vi "Test - Waveform Subtype Enum.vi"() -> ()   [LabVIEW 2013]
uses:
  source/library/Waveform Subtype Enum.ctl
panel:
  out "Null":T1 format="%.0x"
  out "Complex Single":T1 format="%.0x"
  out "Complex Double":T1 format="%.0x"
  out "Complex Extended":T1 format="%.0x"
  out "Analog U8":T1 format="%.0x"
  out "Analog U16":T1 format="%.0x"
  out "Analog U32":T1 format="%.0x"
  out "Analog U64":T1 format="%.0x"
  out "Analog I64":T1 format="%.0x"
  out "Analog I8":T1 format="%.0x"
  out "Analog I16":T1 format="%.0x"
  out "Analog I32":T1 format="%.0x"
  out "Digital Data":T1 format="%.0x"
  out "Digital Waveform":T1 format="%.0x"
  out "Dynamic Data":T1 format="%.0x"
  out "Analog Extended":T1 format="%.0x"
  out "Analog Double":T1 format="%.0x"
  out "Analog Single":T1 format="%.0x"
  out "Timestamp":T1 format="%.0x"
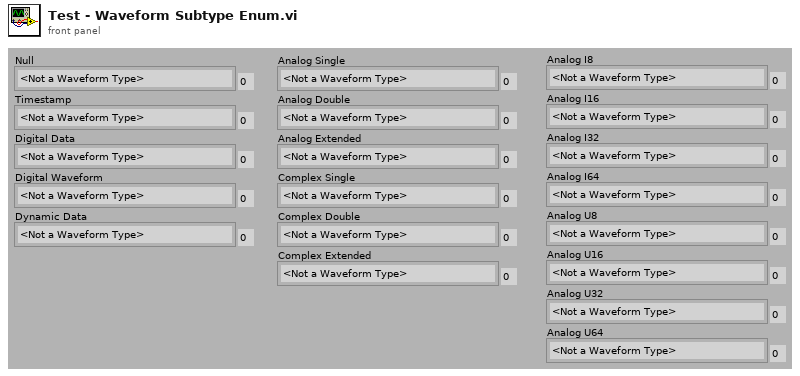
[diagram p1: front panel]
types:
  T1 = typedef "Waveform Subtype Enum.ctl" = enum8{"<Not a Waveform Type>", "0x01", "Analog 16-bit signed", "Analog Double-Precision", "0x04", "Analog Single Precision", "Timestamp", "Digital Data", "Digital Waveform", "Dynamic Data", "Analog Extended-Precision", "Analog 8-bit unsigned", "Analog 16-bit unsigned", "Analog 32-bit unsigned", "Analog 8-bit signed", "Analog 32-bit signed", "Analog Complex Single-Precision", "Analog Complex Double-Precision", "Analog Complex Extended Precision", "Analog 64-bit signed", "Analog 64-bit unsigned"}
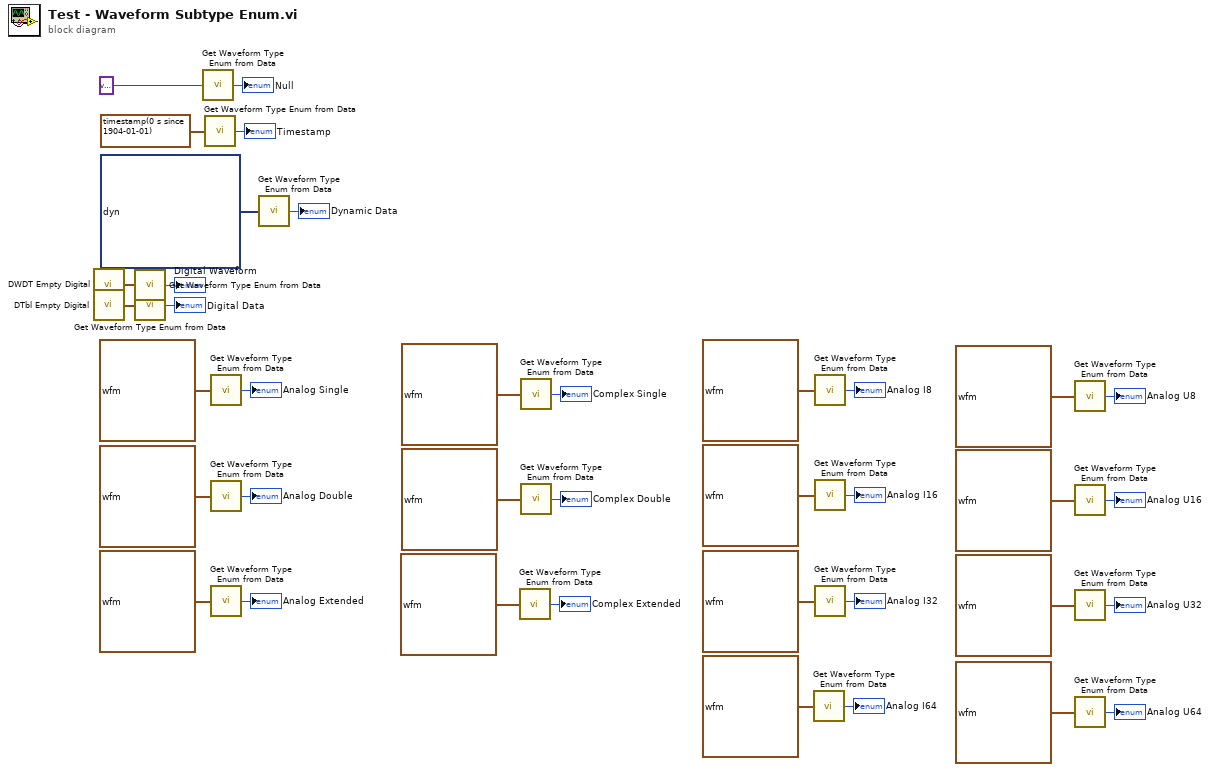
[diagram p0: block diagram]
diagram:
  n1 = call <vilib>:"DWDT Empty Digital.vi"() -> ("digital waveform out"=w27:digitalwaveform)  [unwired: 5 in]
  n2 = call <vilib>:"DTbl Empty Digital.vi"() -> ("digital data"=w25:digitaldata)  [unwired: 5 in]
  n3 = call "Get Waveform Type Enum from Data.vi"("Data"=w27) -> ("Waveform Subtype Enum"=→"Digital Waveform":T1)  [unwired: 4 in]
  n4 = call "Get Waveform Type Enum from Data.vi"("Data"=w25) -> ("Waveform Subtype Enum"=→"Digital Data":T1)  [unwired: 4 in]
  n5 = call "Get Waveform Type Enum from Data.vi"("Data"=variant ("variant")) -> ("Waveform Subtype Enum"=→"Null":T1)  [unwired: 4 in]
  n6 = call "Get Waveform Type Enum from Data.vi"("Data"=timestamp(0 s since 1904-01-01) ("Time Stamp")) -> ("Waveform Subtype Enum"=→"Timestamp":T1)  [unwired: 4 in]
  n7 = call "Get Waveform Type Enum from Data.vi"("Data"=waveform(sgl) {"t0"=timestamp(0 s since 1904-01-01), "dt"=1.0, "Y"=[]} ("waveform")) -> ("Waveform Subtype Enum"=→"Analog Single":T1)  [unwired: 4 in]
  n8 = call "Get Waveform Type Enum from Data.vi"("Data"=waveform(dbl) {"t0"=timestamp(0 s since 1904-01-01), "dt"=1.0, "Y"=[]} ("waveform")) -> ("Waveform Subtype Enum"=→"Analog Double":T1)  [unwired: 4 in]
  n9 = call "Get Waveform Type Enum from Data.vi"("Data"=waveform(ext) {"t0"=timestamp(0 s since 1904-01-01), "dt"=1.0, "Y"=[]} ("waveform")) -> ("Waveform Subtype Enum"=→"Analog Extended":T1)  [unwired: 4 in]
  n10 = call "Get Waveform Type Enum from Data.vi"("Data"=dynamicdata [] ("Waveform Graph")) -> ("Waveform Subtype Enum"=→"Dynamic Data":T1)  [unwired: 4 in]
  n11 = call "Get Waveform Type Enum from Data.vi"("Data"=waveform(cxt) {"t0"=timestamp(0 s since 1904-01-01), "dt"=1.0, "Y"=[]} ("waveform")) -> ("Waveform Subtype Enum"=→"Complex Extended":T1)  [unwired: 4 in]
  n12 = call "Get Waveform Type Enum from Data.vi"("Data"=waveform(csg) {"t0"=timestamp(0 s since 1904-01-01), "dt"=1.0, "Y"=[]} ("waveform")) -> ("Waveform Subtype Enum"=→"Complex Single":T1)  [unwired: 4 in]
  n13 = call "Get Waveform Type Enum from Data.vi"("Data"=waveform(cdb) {"t0"=timestamp(0 s since 1904-01-01), "dt"=1.0, "Y"=[]} ("waveform")) -> ("Waveform Subtype Enum"=→"Complex Double":T1)  [unwired: 4 in]
  n14 = call "Get Waveform Type Enum from Data.vi"("Data"=waveform(i64) {"t0"=timestamp(0 s since 1904-01-01), "dt"=1.0, "Y"=[]} ("waveform")) -> ("Waveform Subtype Enum"=→"Analog I64":T1)  [unwired: 4 in]
  n15 = call "Get Waveform Type Enum from Data.vi"("Data"=waveform(i8) {"t0"=timestamp(0 s since 1904-01-01), "dt"=1.0, "Y"=[]} ("waveform")) -> ("Waveform Subtype Enum"=→"Analog I8":T1)  [unwired: 4 in]
  n16 = call "Get Waveform Type Enum from Data.vi"("Data"=waveform(i16) {"t0"=timestamp(0 s since 1904-01-01), "dt"=1.0, "Y"=[]} ("waveform")) -> ("Waveform Subtype Enum"=→"Analog I16":T1)  [unwired: 4 in]
  n17 = call "Get Waveform Type Enum from Data.vi"("Data"=waveform(i32) {"t0"=timestamp(0 s since 1904-01-01), "dt"=1.0, "Y"=[]} ("waveform")) -> ("Waveform Subtype Enum"=→"Analog I32":T1)  [unwired: 4 in]
  n18 = call "Get Waveform Type Enum from Data.vi"("Data"=waveform(u8) {"t0"=timestamp(0 s since 1904-01-01), "dt"=1.0, "Y"=[]} ("waveform")) -> ("Waveform Subtype Enum"=→"Analog U8":T1)  [unwired: 4 in]
  n19 = call "Get Waveform Type Enum from Data.vi"("Data"=waveform(u16) {"t0"=timestamp(0 s since 1904-01-01), "dt"=1.0, "Y"=[]} ("waveform")) -> ("Waveform Subtype Enum"=→"Analog U16":T1)  [unwired: 4 in]
  n20 = call "Get Waveform Type Enum from Data.vi"("Data"=waveform(u32) {"t0"=timestamp(0 s since 1904-01-01), "dt"=1.0, "Y"=[]} ("waveform")) -> ("Waveform Subtype Enum"=→"Analog U32":T1)  [unwired: 4 in]
  n21 = call "Get Waveform Type Enum from Data.vi"("Data"=waveform(u64) {"t0"=timestamp(0 s since 1904-01-01), "dt"=1.0, "Y"=[]} ("waveform")) -> ("Waveform Subtype Enum"=→"Analog U64":T1)  [unwired: 4 in]
